vi "DSF Pre-Build.vi"   [LabVIEW 2017]
uses:
  Development Tools/Build Automation/Build Automation.lvlib
types:
  T1 = cluster{"Status Message":refnum<data-value>, "Progress":refnum<data-value>, "Stop":refnum<data-value>}
  T2 = enum16{"Share clones between instances", "Preallocate clone for each instance"}
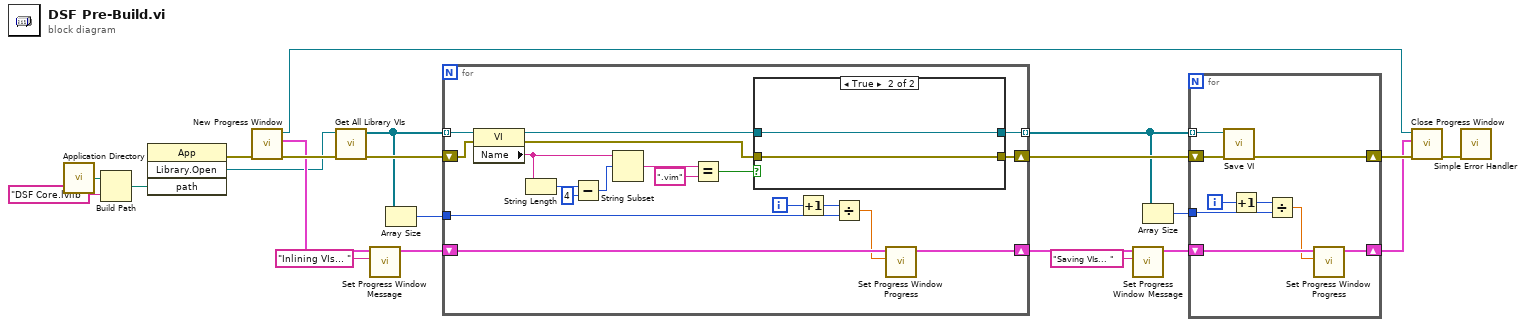
[diagram p0: block diagram]
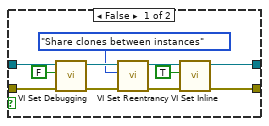
[diagram p2: hidden frame]
diagram:
  n1 = call <vilib>:"Application Directory.vi"() -> ("Application Directory"=w2:path)
  n2 = Build Path(base path=w2, name or relative path="DSF Core.lvlib" ("library name")) -> (appended path=w1:path)
  n3 = invoke class="App" method="Library.Open"("path"=w1) -> (error out=w21:errorcluster, "Open Library"=w9:refnum<vi>)  [unwired: 3 in, 2 out]
  n4 = call "New Progress Window.vi"("error in (no error)"=w21) -> ("error out"=w11:errorcluster, "DVRs"=w10:T1, "VI refnum"=w15:refnum<vi>)  [unwired: 8 in]
  n5 = call "Get All Library VIs.vi"("error in (no error)"=w11, "library ref"=w9) -> ("error out"=w22:errorcluster, "vi refs"=w19:refnum<vi>[])  [unwired: 8 in]
  n6 = call "Set Progress Window Message.vi"("Status Message"="Inlining VIs... " ("data value"), "DVRs in"=w10) -> ("DVRs out"=w17:T1)  [unwired: 8 in, 1 out]
  n7 = Array Size(array=w19) -> (size(s)=w18:i32)
  n8 = for {
    tunnel: w19 -> [w34] mode=indexing
    shift-right: [w35] -> w14
    shift-left: w22 -> [w33]
    tunnel: w18 -> [w25]
    shift-right: [w37] -> w13
    shift-left: w17 -> [w39]
    tunnel: [w36] -> w7 mode=indexing
    i -> [w41]
    n9 = property class="VI"(reference=w34, error in=w33) -> (reference out=w24:refnum<vi>, error out=w32:errorcluster, "Name"=w31:string)
    n10 = String Length(string=w31) -> (length=w30:i32)
    n11 = Subtract(x=w30, y=4) -> (x-y=w23:i32)
    n12 = String Subset(string=w31, offset (0)=w23) -> (substring=w28:string)  [unwired: 1 in]
    n13 = Equal?(x=w28, y=".vim") -> (x = y?=w26:bool)
    n14 = case shown="True" w26 {
      tunnel: [w45 w53] -> w36
      tunnel: [w42 w54] -> w35
      tunnel: w32 -> [w44 w54]
      tunnel: w24 -> [w43 w53]
      frame False {
        n15 = call "VI Set Debugging.vi"("error in (no error)"=w44, "Allow Debugging"=FALSE, "vi ref in"=w43) -> ("error out"=w50:errorcluster, "vi ref out"=w51:refnum<vi>)  [unwired: 7 in]
        n16 = call "VI Set Reentrancy.vi"("error in (no error)"=w50, "Reentrancy Type"=T2."Share clones between instances", "vi ref in"=w51) -> ("error out"=w48:errorcluster, "vi ref out"=w49:refnum<vi>)  [unwired: 7 in]
        n17 = call "VI Set Inline.vi"("error in (no error)"=w48, "Inline VI"=TRUE, "vi ref in"=w49) -> ("error out"=w42:errorcluster, "vi ref out"=w45:refnum<vi>)  [unwired: 7 in]
      }
      frame True {
      }
    }
    n18 = Increment(x=w41) -> (x+1=w40:i32)
    n19 = Divide(x=w40, y=w25) -> (x/y=w38:dbl)
    n20 = call "Set Progress Window Progress.vi"("Progress"=w38, "DVRs in"=w39) -> ("DVRs out"=w37:T1)  [unwired: 8 in, 1 out]
  }
  n21 = call "Set Progress Window Message.vi"("Status Message"="Saving VIs... ", "DVRs in"=w13) -> ("DVRs out"=w8:T1)  [unwired: 8 in, 1 out]
  n22 = Array Size(array=w7) -> (size(s)=w6:i32)
  n23 = for {
    shift-right: [w61] -> w5
    shift-left: w14 -> [w63]
    tunnel: w7 -> [w62] mode=indexing
    shift-right: [w55] -> w4
    shift-left: w8 -> [w57]
    tunnel: w6 -> [w59]
    i -> [w58]
    n24 = call "Save VI.vi"("error in (no error)"=w63, "vi ref in"=w62) -> ("error out"=w61:errorcluster)  [unwired: 8 in, 1 out]
    n25 = Increment(x=w58) -> (x+1=w60:i32)
    n26 = Divide(x=w60, y=w59) -> (x/y=w56:dbl)
    n27 = call "Set Progress Window Progress.vi"("Progress"=w56, "DVRs in"=w57) -> ("DVRs out"=w55:T1)  [unwired: 8 in, 1 out]
  }
  n28 = call "Close Progress Window.vi"("error in (no error)"=w5, "DVRs in"=w4, "VI refnum"=w15) -> ("error out"=w16:errorcluster)  [unwired: 8 in]
  n29 = call <vilib>:"Simple Error Handler.vi"("error in (no error)"=w16) -> ()  [unwired: 4 in, 5 out]
